vi "Powershell Test.vi"() -> ()   [LabVIEW 2019]
panel:
  in  "StdIn":string="ping -n 3 127.0.0.1\nWrite-Host \"hello\"\nCopy-Item -Path \"C:\\intentionally\\invalid\\path\" -Destination \"C:\\another\\intentionally\\invalid\\path\"\nWrite-Error \"Another intentional error\"\nexit"
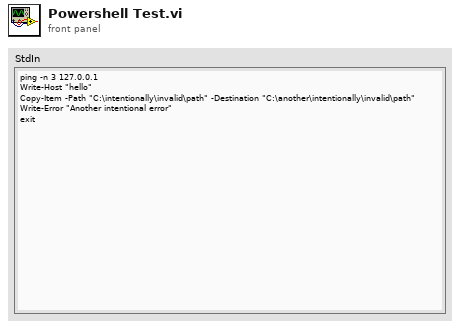
[diagram p1: front panel]
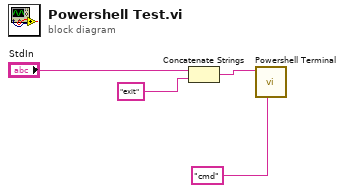
[diagram p0: block diagram]
diagram:
  n1 = Concatenate Strings("StdIn", "exit" ("string")) -> (w2:string)
  n2 = call "Powershell Terminal.vi"("command line"="cmd", "StdIn"=w2) -> ()  [unwired: 7 in, 3 out]
